vi "Synchronize Control VI.vi"(8 "error in (no error)":errorcluster, 10 "Control Destination":path, 11 "Control in":refnum<class "Control.lvclass">) -> (0 "error out":errorcluster, 3 "Control out":refnum<class "Control.lvclass">)   [LabVIEW 2013, in "uitools_Control.lvlib" / "Control.lvclass"]
uses:
  Control.lvclass
  <vilib>/Utility/miscctls.llb/LVFontTypeDef.ctl
  <vilib>/Utility/miscctls.llb/LVPositionTypeDef.ctl
  <userlib>/BitMan/BitMap class/BitMap.lvclass
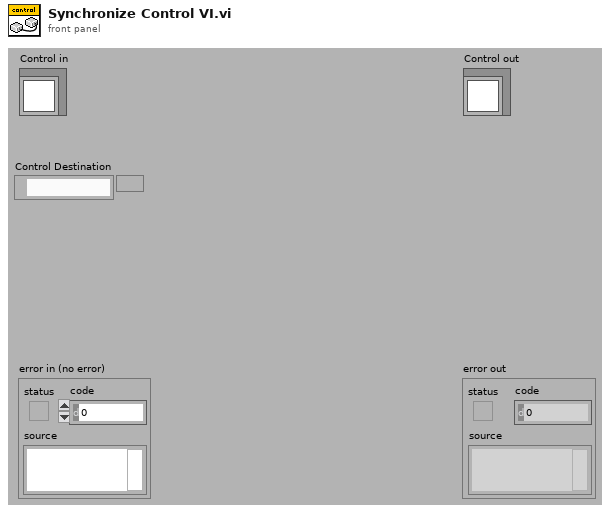
[diagram p1: front panel]
types:
  T1 = typedef "LVFontTypeDef.ctl" = cluster{"Font Name":string, "Size":u16, "Bold":bool, "Italic":bool, "Underline":bool, "Strikeout":bool, "Color":u32}
  T2 = typedef "LVPositionTypeDef.ctl" = cluster{"Left":i32, "Top":i32}
  T3 = typedef "imagedata.ctl" = cluster{"image type":i32, "image depth":i32, "image":u8[], "mask":u8[], "colors":u32[], "Rectangle":cluster{"left":i16, "top":i16, "right":i16, "bottom":i16}}
  T4 = typedef "uitools_Control.lvlib/Control.lvclass/BX.Orientation__LCR _Modified.ctl" = u8
  T5 = cluster{"left":i16, "top":i16, "right":i16, "bottom":i16}
  T6 = typedef "uitools_Control.lvlib/Control.lvclass/_ui_tools_font.ctl" = cluster{"Font Name:":string, "Size":i16, "Strikeout?":bool, "Italic?":bool, "Underline?":bool, "Outline?":bool, "Shadow?":bool, "Bold?":bool}
  T7 = typedef "uitools_Control.lvlib/Control.lvclass/TypeDef_Action.ctl" = u16
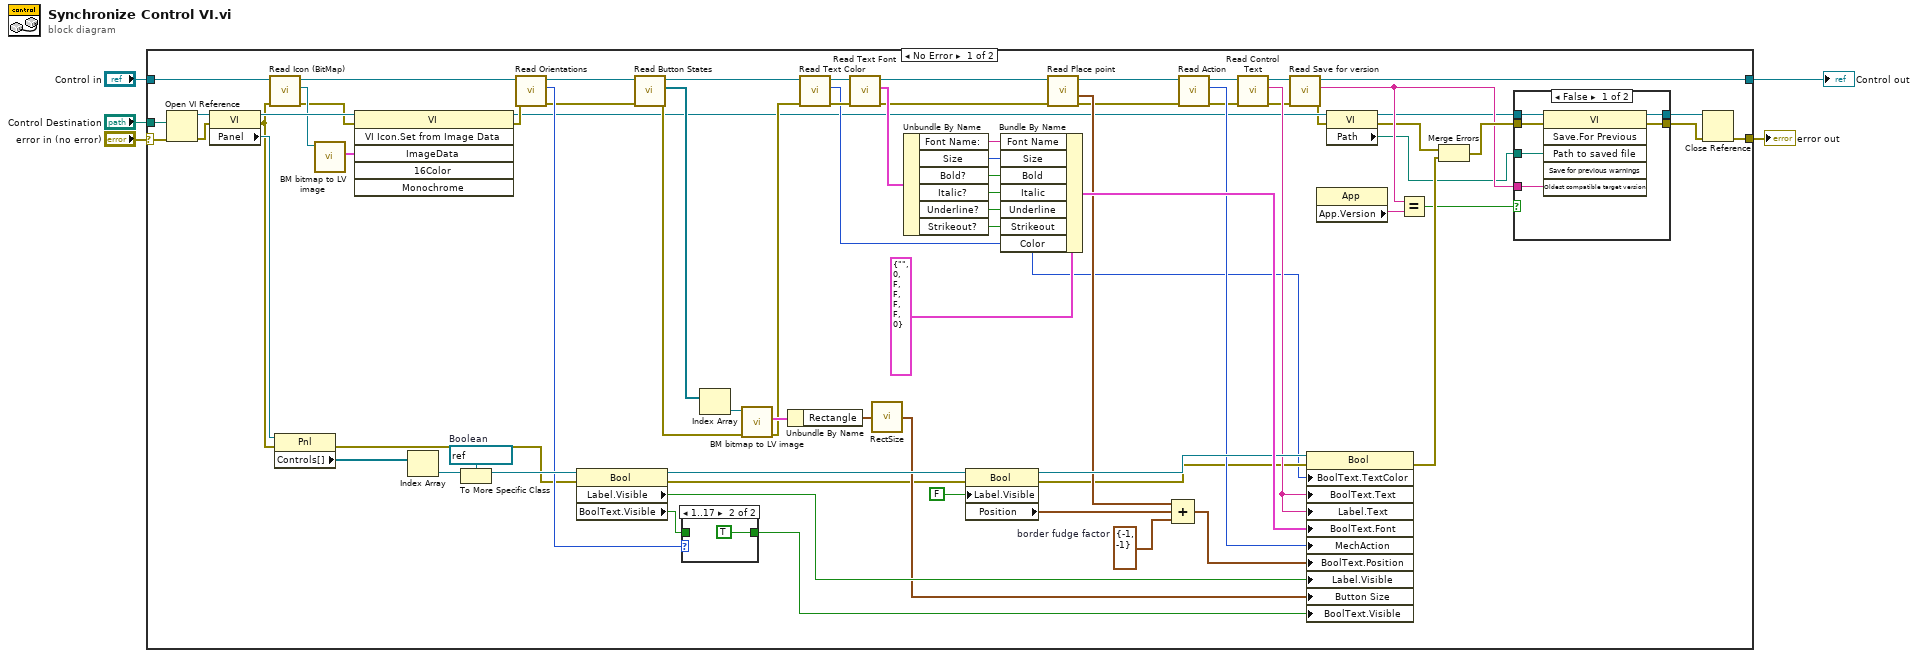
[diagram p0: block diagram]
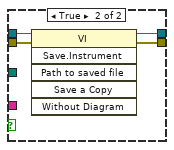
[diagram p2: hidden frame]
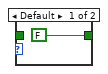
[diagram p3: hidden frame]
diagram:
  n1 = case shown="No Error" "error in (no error)" {
    selector: "error in (no error)" -> [w73 w96]
    tunnel: [w74 w96] -> w4
    tunnel: [w15 w95] -> w2
    tunnel: "Control in" -> [w47 w95]
    tunnel: "Control Destination" -> [w76 _]
    frame No Error {
      w17 = T2 {"Left"=-1, "Top"=-1}  # border fudge factor
      w79 = refnum<vi> refnum  # Boolean
      n2 = Open VI Reference(vi path=w76, error in (no error)=w73) -> (vi reference=w82:refnum<vi>, error out=w72:errorcluster)  [unwired: 4 out]
      n3 = property class="VI"(reference=w82, error in=w72) -> (reference out=w60:refnum<vi>, error out=w30:errorcluster, "Panel"=w81:refnum<vi>)
      n4 = call-dynamic "Read Icon (BitMap).vi"("error in (no error)"=w30, "Control in"=w47) -> ("error out"=w35:errorcluster, "Icon (BitMap) False"=w45:refnum<class "BitMap.lvclass">, "Control out"=w46:refnum<class "Control.lvclass">)  [unwired: 7 out]
      n5 = property class="Pnl"(reference=w81, error in=w30) -> (error out=w29:errorcluster, "Controls[]"=w80:refnum<vi>[])  [unwired: 1 out]
      n6 = call <userlib>:"BM bitmap to LV image.vi"("BitMap in"=w45) -> ("LV image data"=w61:T3)  [unwired: 2 in, 8 out]
      n7 = invoke class="VI" method="VI Icon.Set from Image Data"(reference=w60, error in=w35, "ImageData"=w61) -> (reference out=w10:refnum<vi>, error out=w34:errorcluster)  [unwired: 3 in, 4 out]
      n8 = Index Array(array=w80) -> (element=w78:refnum<vi>)  [unwired: 1 in]
      n9 = To More Specific Class(target class=w79, reference=w78) -> (specific class reference=w55:refnum<vi>)  [unwired: 1 in, 1 out]
      n10 = call-dynamic "Read Orientations.vi"("error in (no error)"=w34, "Control in"=w46) -> ("error out"=w33:errorcluster, "Orientations"=w51:T4, "Control out"=w41:refnum<class "Control.lvclass">)  [unwired: 7 out]
      n11 = property class="Bool"(reference=w55, error in=w29) -> (reference out=w54:refnum<vi>, error out=w27:errorcluster, "Label.Visible"=w50:bool, "BoolText.Visible"=w49:bool)
      n12 = call-dynamic "Read Button States.vi"("error in (no error)"=w33, "Control in"=w41) -> ("error out"=w28:errorcluster, "Button States"=w40:refnum<class "BitMap.lvclass">[], "Control out"=w22:refnum<class "Control.lvclass">)  [unwired: 7 out]
      n13 = case shown="1..17" w51 {
        tunnel: [FALSE TRUE] -> w48
        tunnel: w49 -> [_ _]
        frame Default {
        }
        frame 1..17 {
        }
      }
      n14 = Index Array(array=w40) -> (element=w53:refnum<class "BitMap.lvclass">)  [unwired: 1 in]
      n15 = call <userlib>:"BM bitmap to LV image.vi"("error in (no error)"=w28, "BitMap in"=w53) -> ("error out"=w20:errorcluster, "LV image data"=w52:T3)  [unwired: 1 in, 7 out]
      n16 = Unbundle By Name(w52) -> ("Rectangle"=w44:T5)
      n17 = call-dynamic "Read Text Color.vi"("error in (no error)"=w20, "Control.lvclass in"=w22) -> ("error out"=w19:errorcluster, "Text Color"=w18:u32, "Control.lvclass out"=w21:refnum<class "Control.lvclass">)  [unwired: 7 out]
      n18 = call-dynamic "Read Text Font.vi"("error in (no error)"=w19, "Control in"=w21) -> ("error out"=w32:errorcluster, "Font"=w71:T6, "Control out"=w36:refnum<class "Control.lvclass">)  [unwired: 7 out]
      n19 = call <vilib>:"RectSize.vi"("rect"=w44) -> ("point"=w43:cluster{"x":i16, "y":i16})
      n20 = Unbundle By Name(w71) -> ("Font Name:"=w69:string, "Size"=w67:i16, "Bold?"=w66:bool, "Italic?"=w65:bool, "Underline?"=w64:bool, "Strikeout?"=w63:bool)
      n21 = property class="Bool"(reference=w54, error in=w27, "Label.Visible"=FALSE) -> (reference out=w62:refnum<vi>, error out=w26:errorcluster, "Position"=w58:T2)
      n22 = Bundle By Name(cluster=T1 {"Font Name"="", "Size"=0, "Bold"=FALSE, "Italic"=FALSE, "Underline"=FALSE, "Strikeout"=FALSE, "Color"=0} ("Boolean Text.Font"), "Font Name"=w69, "Size"=w67, "Bold"=w66, "Italic"=w65, "Underline"=w64, "Strikeout"=w63, "Color"=w18) -> (w68:T1)
      n23 = call-dynamic "Read Place point.vi"("error in (no error)"=w32, "Control in"=w36) -> ("error out"=w31:errorcluster, "Text Point"=w59:cluster{"x":i32, "y":i32}, "Control out"=w39:refnum<class "Control.lvclass">)  [unwired: 7 out]
      n24 = Compound Arithmetic op=ADD(w59, w58, w17) -> (w56:T2)
      n25 = call-dynamic "Read Action.vi"("error in (no error)"=w31, "Control in"=w39) -> ("error out"=w25:errorcluster, "Action"=w37:T7, "Control out"=w38:refnum<class "Control.lvclass">)  [unwired: 7 out]
      n26 = call-dynamic "Read Control Text.vi"("error in (no error)"=w25, "Control in"=w38) -> ("error out"=w14:errorcluster, "Control Text"=w42:string, "Control out"=w16:refnum<class "Control.lvclass">)  [unwired: 7 out]
      n27 = call-dynamic "Read Save for version.vi"("error in (no error)"=w14, "Control.lvclass in"=w16) -> ("error out"=w7:errorcluster, "Save for version"=w11:string, "Control.lvclass out"=w15:refnum<class "Control.lvclass">)  [unwired: 7 out]
      n28 = property class="Bool"(reference=w62, error in=w26, "BoolText.TextColor"=w18, "BoolText.Text"=w42, "Label.Text"=w42, "BoolText.Font"=w68, "MechAction"=w37, "BoolText.Position"=w56, "Label.Visible"=w50, "Button Size"=w43, "BoolText.Visible"=w48) -> (error out=w24:errorcluster)  [unwired: 1 out]
      n29 = property class="App"() -> ("App.Version"=w13:string)  [unwired: 2 in, 2 out]
      n30 = property class="VI"(reference=w10, error in=w7) -> (reference out=w9:refnum<vi>, error out=w6:errorcluster, "Path"=w8:path)
      n31 = Equal?(x=w11, y=w13) -> (x = y?=w12:bool)
      n32 = Merge Errors(w6, w24) -> (w23:errorcluster)
      n33 = case shown="False" w12 {
        tunnel: [w87 w92] -> w77
        tunnel: [w85 w91] -> w75
        tunnel: w9 -> [w88 w90]
        tunnel: w23 -> [w84 w89]
        tunnel: w11 -> [w86 _]
        tunnel: w8 -> [w83 _]
        frame False {
          n34 = invoke class="VI" method="Save.For Previous"(reference=w88, error in=w84, "Path to saved file"=w83, "Oldest compatible target version"=w86) -> (reference out=w87:refnum<vi>, error out=w85:errorcluster)  [unwired: 2 in, 4 out]
        }
        frame True {
          n35 = invoke class="VI" method="Save.Instrument"(reference=w90, error in=w89) -> (reference out=w92:refnum<vi>, error out=w91:errorcluster)  [unwired: 4 in, 4 out]
        }
      }
      n36 = Close Reference(reference=w77, error in (no error)=w75) -> (error out=w74:errorcluster)
    }
    frame Error {
    }
  }
  "error out" <- w4
  "Control out" <- w2
